vi "Rogowski_Coil_Imon.vi"(4 "Ref_Freq":dbl=25000.0, 6 "RefGain":dbl=10.07, 10 "CurrentFreq":dbl=50000.0) -> (2 "x*y":dbl=5.035)   [LabVIEW 2021]
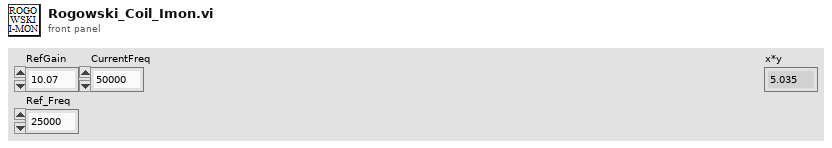
[diagram p1: front panel]
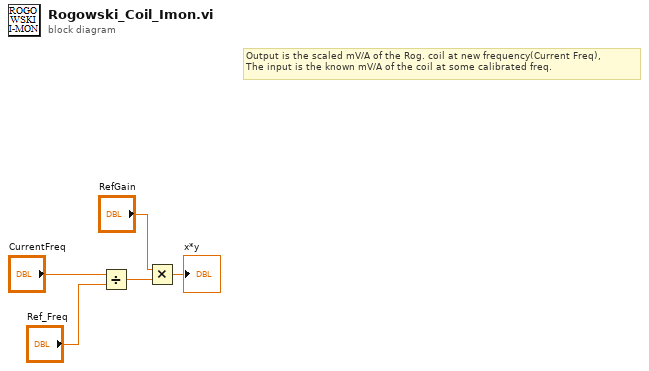
[diagram p0: block diagram]
diagram:
  # "Output is the scaled mV/A of the Rog. coil at new frequency(Current Freq),\nThe input is the known mV/A of the coil at some calibrated freq."
  n1 = Divide(x="CurrentFreq", y="Ref_Freq") -> (x/y=w4:dbl)
  n2 = Multiply(x="RefGain", y=w4) -> (x*y=→"x*y":dbl)
